vi "Delete Item From Listbox.vi"(0 "Display State In":T1, 5 "Item to Delete":string, 9 "Container State":T2, 11 "error in (no error)":errorcluster) -> (4 "Display State Out":T1, 6 "Deleted Item":string, 8 "Invalid Item":bool, 15 "error out":errorcluster)   [LabVIEW 2011, in "X Listbox-Solution.xctl"]
doc: "This is a method for the X Listbox. Details about implementation can be found in the course manual.\n\nAAL 9/09"
uses:
  X Listbox-Solution.xctl
  <vilib>/_xctls/Container State.ctl
  Abilities/X Listbox State.ctl
  <vilib>/_xctls/XControlSupport.lvlib
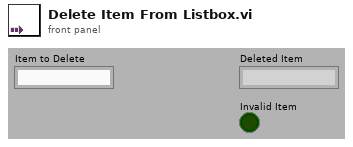
[diagram p1: front panel]
types:
  T1 = typedef "X Listbox-Solution.xctl/X Listbox State.ctl" = cluster{"# Items":i32, "Names":string[]}
  T2 = typedef "XControlSupport.lvlib/Container State.ctl" = cluster{"Indicator?":bool, "Run Mode?":bool, " Refnum":refnum<vi>}
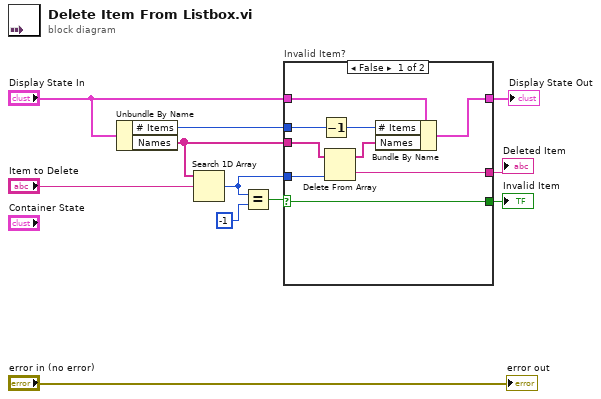
[diagram p0: block diagram]
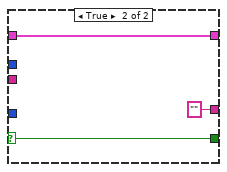
[diagram p2: hidden frame]
diagram:
  n1 = Unbundle By Name("Display State In") -> ("# Items"=w6:i32, "Names"=w5:string[])
  n2 = Search 1D Array(1D array=w5, element="Item to Delete") -> (index of element=w4:i32)  [unwired: 1 in]
  n3 = Equal?(x=w4, y=-1) -> (x = y?=w3:bool)
  n4 = case "Invalid Item?" shown="False" w3 {
    selector: w3 -> [w13 w22]
    tunnel: "Display State In" -> [w20 w23]
    tunnel: [w19 w23] -> w7
    tunnel: w6 -> [w18 _]
    tunnel: w5 -> [w16 _]
    tunnel: w4 -> [w15 _]
    tunnel: [w13 w22] -> w2
    tunnel: [w12 "" ("String")] -> w1
    frame False {
      n5 = Decrement(x=w18) -> (x-1=w17:i32)
      n6 = Delete From Array(array=w16, index=w15) -> (deleted portion=w12:string, array with subset deleted=w14:string[])  [unwired: 1 in]
      n7 = Bundle By Name(cluster=w20, "# Items"=w17, "Names"=w14) -> (w19:T1)
    }
    frame True {
    }
  }
  "Display State Out" <- w7
  "Invalid Item" <- w2
  "Deleted Item" <- w1
  "error out" <- "error in (no error)"
